vi "Amplitude Set.vi"(6 "Update":bool=TRUE, 7 "Amplitude":dbl format="%#_13g", 8 "error in (no error)":errorcluster, 9 "node":i32, 10 "idxChannel":i32, 11 "hdwf":i32) -> (0 "error out":errorcluster, 1 "func_out":i32, 5 "Amp Out":dbl)   [LabVIEW 2024, in "AD2 DLL.lvlib"]
uses:
  AD2 DLL.lvlib
  <vilib>/Digilent/AD2 Toolkit/AD2.lvlib
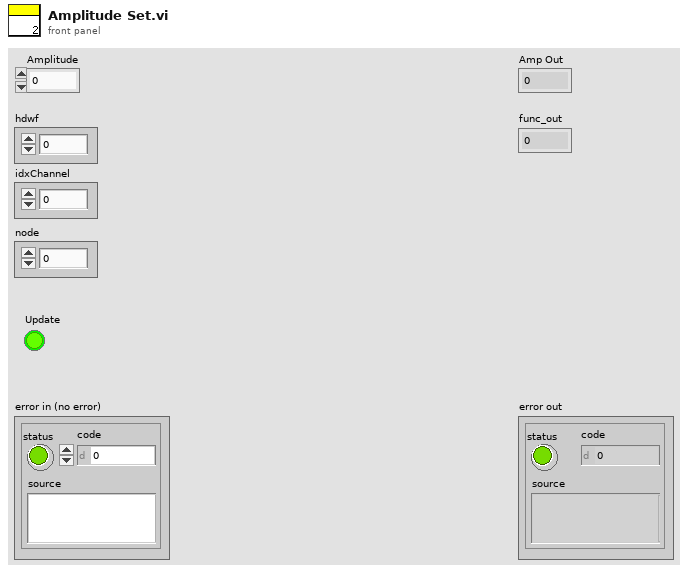
[diagram p1: front panel]
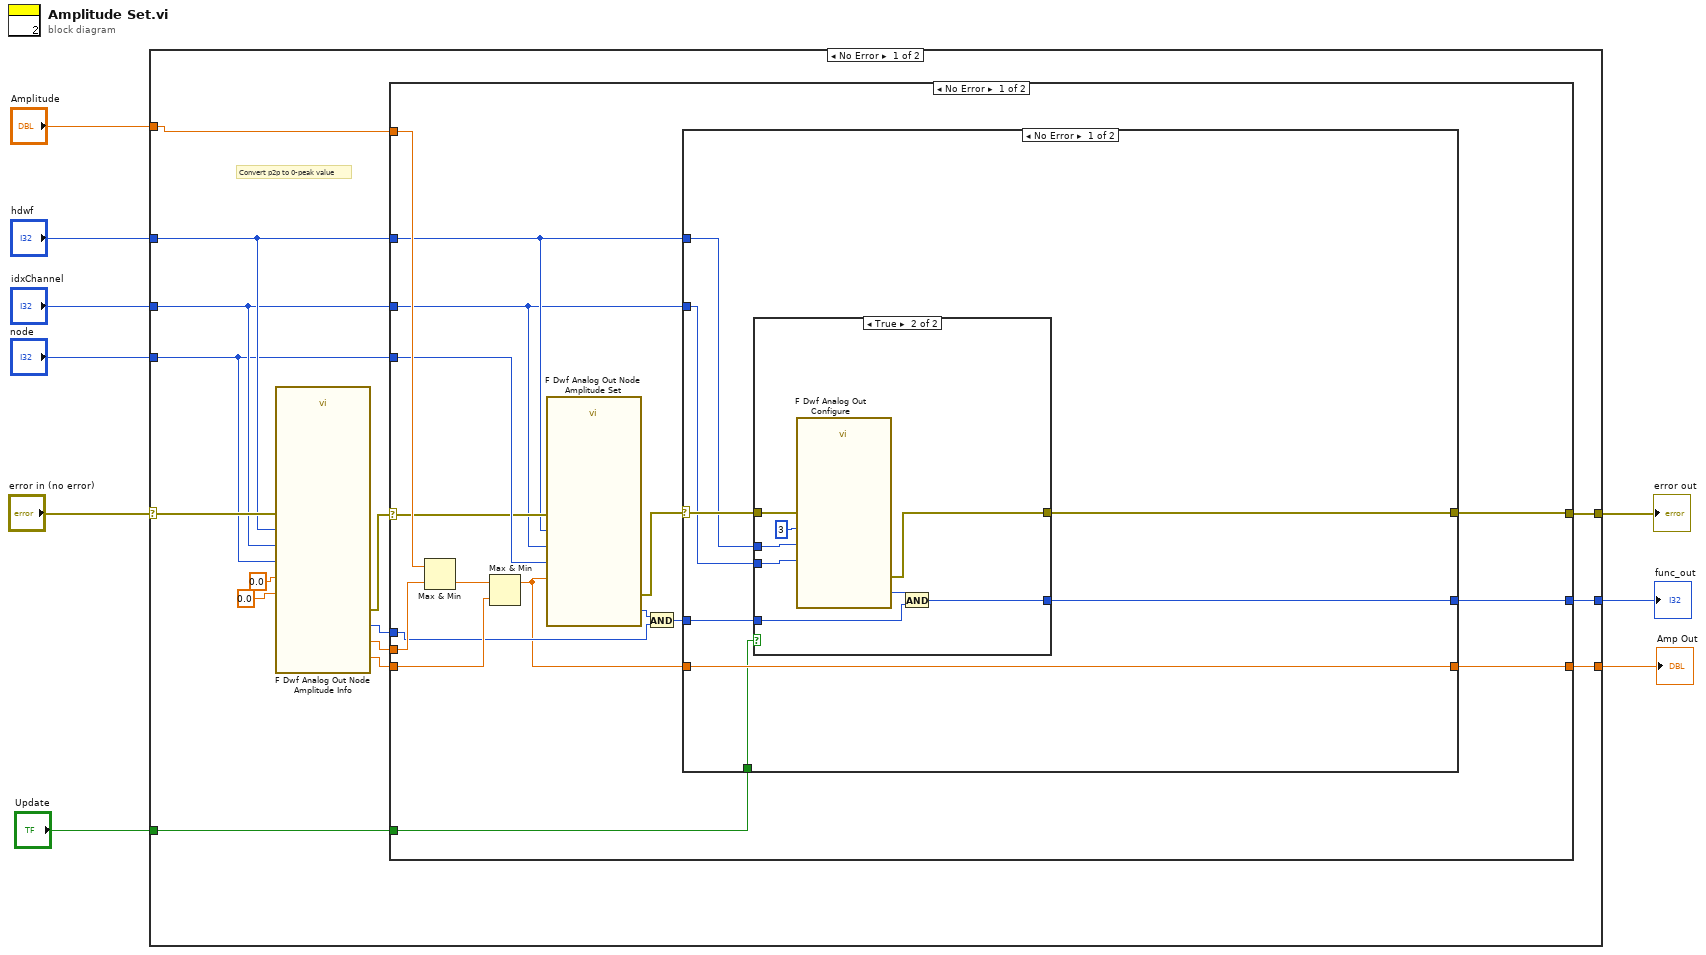
[diagram p0: block diagram]
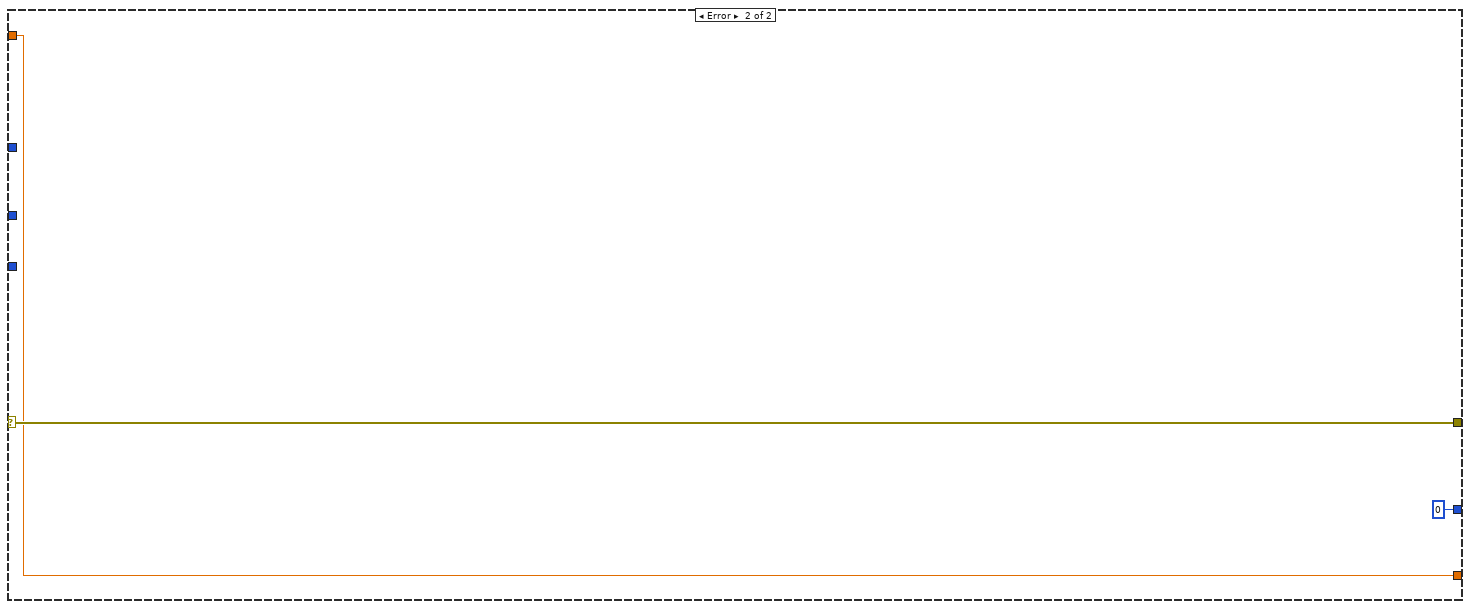
[diagram p5: hidden frame]
diagram:
  n1 = case shown="No Error" "error in (no error)" {
    selector: "error in (no error)" -> [w24 w68]
    tunnel: [w18 w68] -> w9
    tunnel: "hdwf" -> [w17 _]
    tunnel: "idxChannel" -> [w16 _]
    tunnel: "node" -> [w15 _]
    tunnel: "Amplitude" -> [w21 w66]
    tunnel: [w12 0] -> w3
    tunnel: [w11 w66] -> w2
    tunnel: "Update" -> [w10 _]
    frame No Error {
      # "Convert p2p to 0-peak value"
      n2 = call <vilib>:"F Dwf Analog Out Node Amplitude Info.vi"("pMax"=0.0, "pMin"=0.0, "error in (no error)"=w24, "node"=w15, "idxChannel"=w16, "hdwf"=w17) -> ("error out"=w14:errorcluster, "function return"=w13:i32, "pMax out"=w20:dbl, "pMin out"=w19:dbl)  [unwired: 2 in]
      n3 = case shown="No Error" w14 {
        selector: w14 -> [w36 w65]
        tunnel: w21 -> [w41 w63]
        tunnel: w20 -> [w40 _]
        tunnel: w19 -> [w38 _]
        tunnel: [w34 w65] -> w18
        tunnel: w17 -> [w33 _]
        tunnel: w16 -> [w32 _]
        tunnel: w15 -> [w37 _]
        tunnel: w13 -> [w30 w64]
        tunnel: [w28 w64] -> w12
        tunnel: [w26 w63] -> w11
        tunnel: w10 -> [w25 _]
        frame No Error {
          n4 = Max & Min(x=w41, y=w40) -> (min(x,y)=w39:dbl)  [unwired: 1 out]
          n5 = Max & Min(x=w39, y=w38) -> (max(x,y)=w27:dbl)  [unwired: 1 out]
          n6 = call <vilib>:"F Dwf Analog Out Node Amplitude Set.vi"("vAmplitude"=w27, "error in (no error)"=w36, "node"=w37, "idxChannel"=w32, "hdwf"=w33) -> ("error out"=w35:errorcluster, "function return"=w31:i32)  [unwired: 5 in]
          n7 = And(x=w31, y=w30) -> (x .and. y?=w29:i32)
          n8 = case shown="No Error" w35 {
            selector: w35 -> [w49 w62]
            tunnel: [w46 w62] -> w34
            tunnel: w33 -> [w48 _]
            tunnel: w32 -> [w47 _]
            tunnel: w29 -> [w45 w61]
            tunnel: [w44 w61] -> w28
            tunnel: w27 -> [w43 w60]
            tunnel: [w43 w60] -> w26
            tunnel: w25 -> [w42 _]
            frame No Error {
              n9 = case shown="True" w42 {
                tunnel: w49 -> [w51 w59]
                tunnel: w48 -> [_ w57]
                tunnel: w47 -> [_ w56]
                tunnel: [w51 w55] -> w46
                tunnel: w45 -> [w50 w53]
                tunnel: [w50 w52] -> w44
                frame False {
                }
                frame True {
                  n10 = call <vilib>:"F Dwf Analog Out Configure.vi"("error in (no error)"=w59, "fStart"=3, "idxChannel"=w56, "hdwf"=w57) -> ("error out"=w55:errorcluster, "function return"=w54:i32)  [unwired: 6 in]
                  n11 = And(x=w54, y=w53) -> (x .and. y?=w52:i32)
                }
              }
            }
            frame Error {
            }
          }
        }
        frame Error {
        }
      }
    }
    frame Error {
    }
  }
  "error out" <- w9
  "func_out" <- w3
  "Amp Out" <- w2
